vi "Write.vi"(8 "error in (no error)":errorcluster, 10 "write buffer":string, 11 "ArduinoAIReal in":refnum<class "Arduino.lvclass">) -> (0 "error out":errorcluster, 3 "ArduinoAIReal out":refnum<class "Arduino.lvclass">)   [LabVIEW 2020, in "Arduino.lvlib" / "Arduino.lvclass"]
uses:
  Arduino.lvclass
  Arduino.lvclass/Arduino.ctl
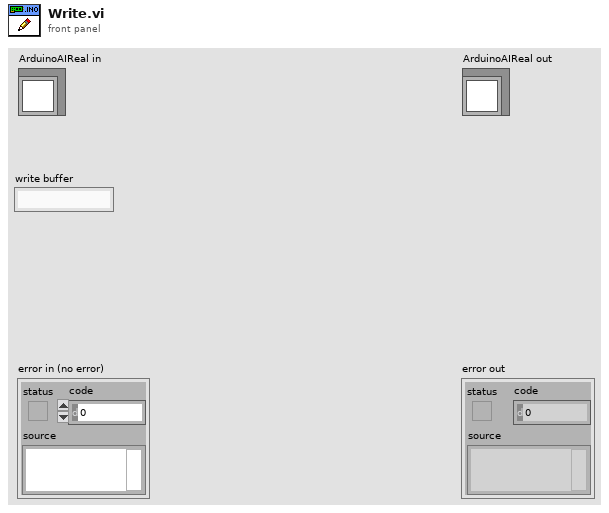
[diagram p1: front panel]
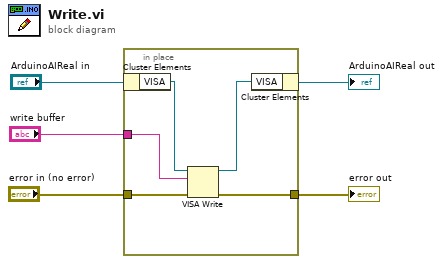
[diagram p0: block diagram]
diagram:
  n1 = in-place {
    in-place-border: [w10] -> w5
    in-place-border: "error in (no error)" -> [w9]
    in-place-border: "write buffer" -> [w6]
    n2 = in-place-cluster #1("ArduinoAIReal in") -> ("VISA"=w8:refnum<visa-resource-name>)
    n3 = VISA Write(VISA resource name=w8, write buffer=w6, error in (no error)=w9) -> (VISA resource name out=w7:refnum<visa-resource-name>, error out=w10:errorcluster)  [unwired: 1 out]
    n4 = in-place-cluster #1("VISA"=w7) -> (→"ArduinoAIReal out":refnum<class "Arduino.lvclass">)
  }
  "error out" <- w5
